vi "Acquire.vi"(8 "error in (no error)":errorcluster, 9 "DataNotifier":refnum<notifier>[](array[refnum]), 10 "DataQueues":refnum<queue>[](array[refnum]), 11 "Config In":T1 {"Hardware Configuration"."Lasers Configuration"."SettingValues"."785 Power" format="%.1f"; "Hardware Configuration"."Lasers Configuration"."SettingValues"."647 Power" format="%.1f"; "Hardware Configuration"."Lasers Configuration"."SettingValues"."561 Power" format="%.1f"; "Hardware Configuration"."Lasers Configuration"."SettingValues"."532 Power" format="%.1f"; "Hardware Configuration"."Lasers Configuration"."SettingValues"."488 Power" format="%.1f"; "Hardware Configuration"."Lasers Configuration"."SettingValues"."405 Power" format="%.1f"}) -> (0 "error out":errorcluster, 3 "Config Out":T1 {"Hardware Configuration"."Lasers Configuration"."SettingValues"."785 Power" format="%.1f"; "Hardware Configuration"."Lasers Configuration"."SettingValues"."647 Power" format="%.1f"; "Hardware Configuration"."Lasers Configuration"."SettingValues"."561 Power" format="%.1f"; "Hardware Configuration"."Lasers Configuration"."SettingValues"."532 Power" format="%.1f"; "Hardware Configuration"."Lasers Configuration"."SettingValues"."488 Power" format="%.1f"; "Hardware Configuration"."Lasers Configuration"."SettingValues"."405 Power" format="%.1f"})   [LabVIEW 2019, in "Acquisition.lvlib"]
doc: "Perform the acquisition. Replace the contents of this diagram with calls to acquisition hardware."
uses:
  Acquisition.lvlib
  Settings/Settings.ctl
  HardwareAdapter/Support/Hardware Configuration.ctl
  HardwareAdapter/Support/Camera Configuration.ctl
  D:/SDK/PMQI-LabViewSamples/Examples/Dependencies/PVCamNET.dll
  <vilib>/userdefined/High Color/IMAQdx.ctl
  E:/DevHardSoftware/MMicroscopy/HardwareAdapter/Lasers/Dependencies/Oxxius_Boxx.dll
  HardwareAdapter/Lasers/Dependencies/Oxxius_Boxx.dll
  Logging/Logging Configuration.ctl
  controls/UI Configuration.ctl
  Global.vi
  Logging/Logging.lvlib
  Settings/Settings.lvlib
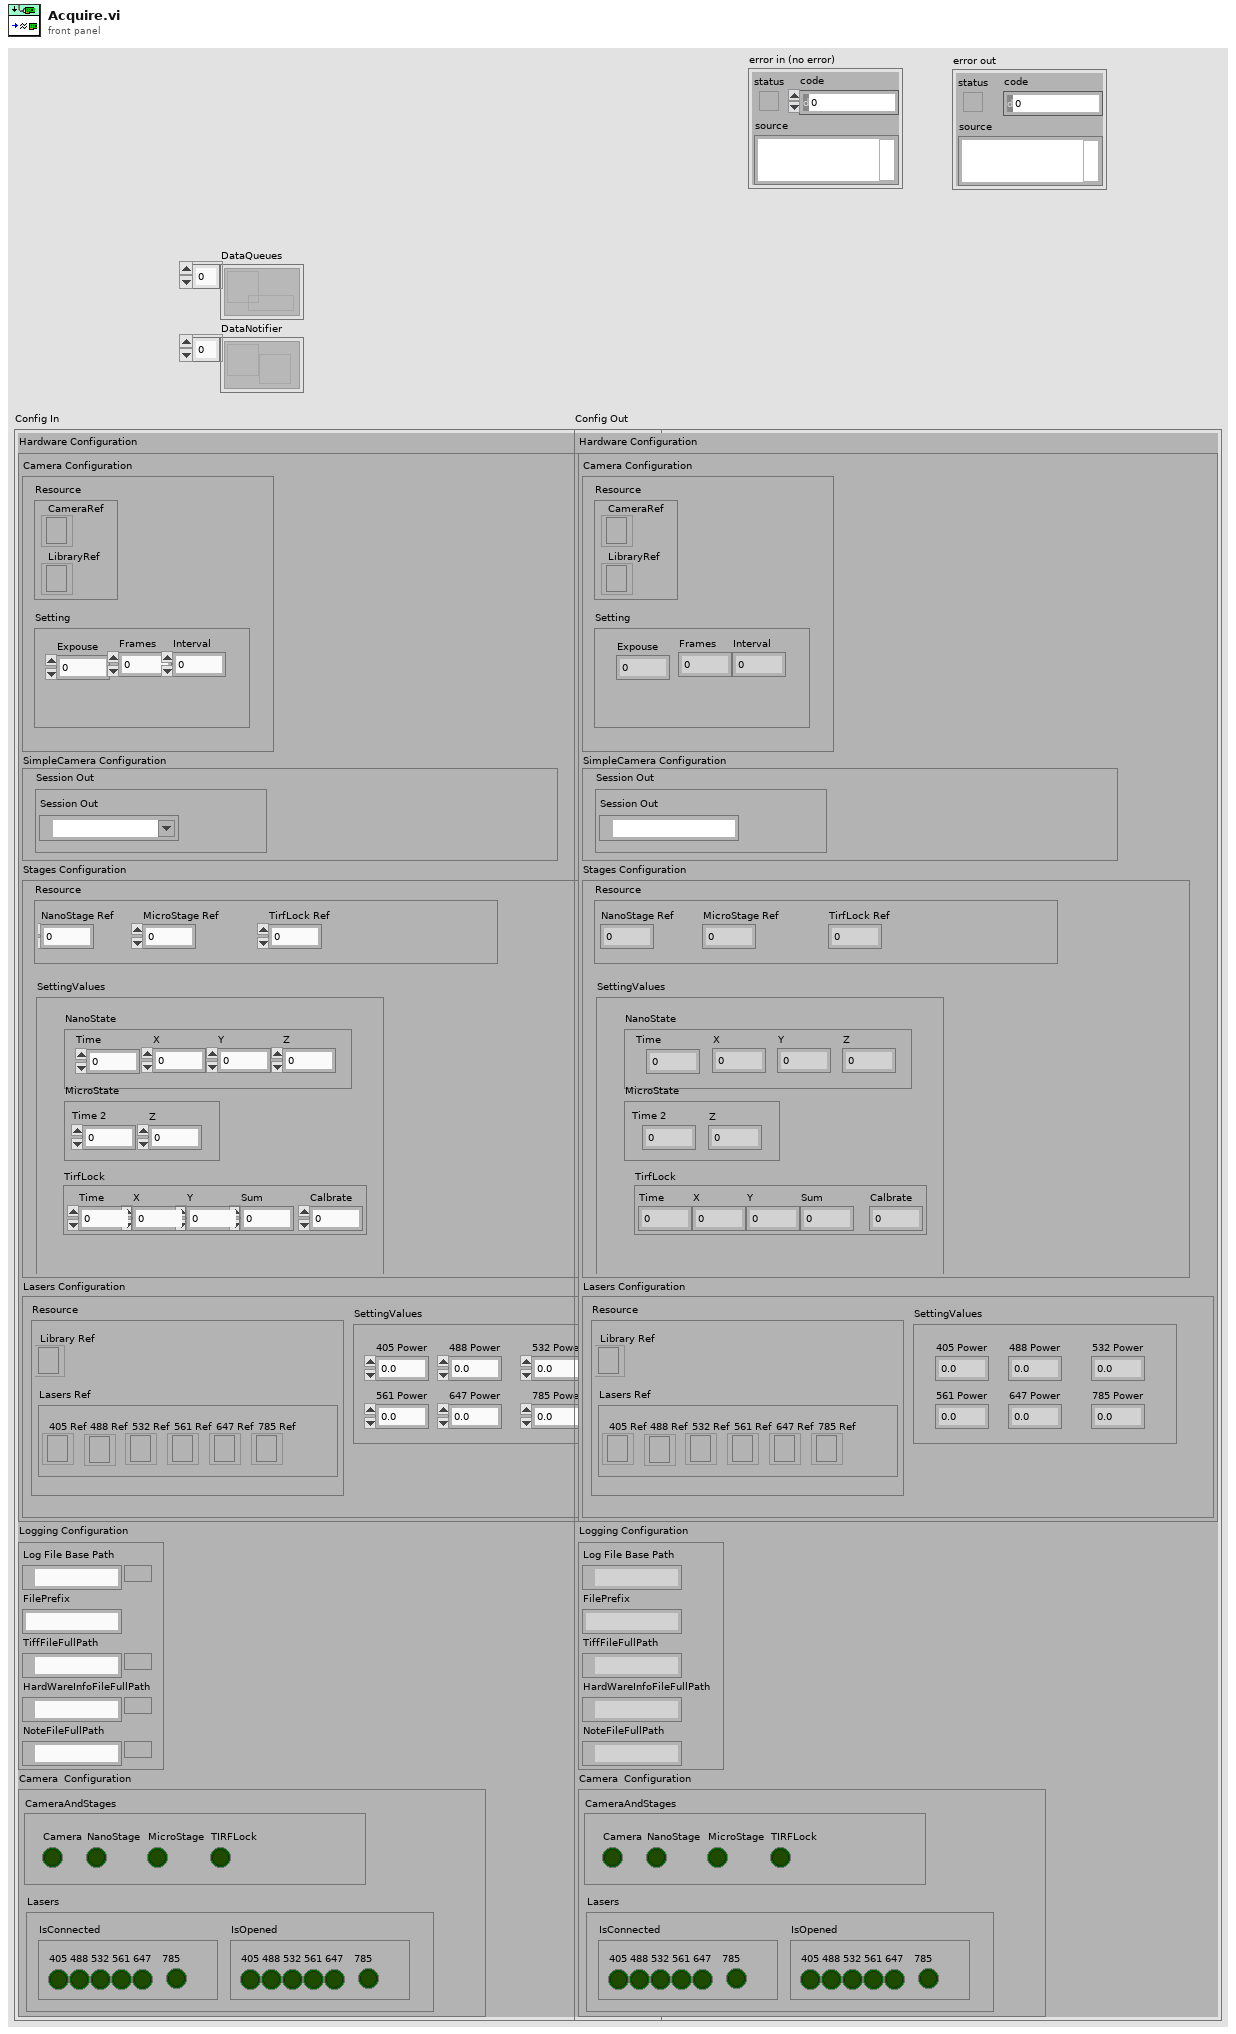
[diagram p1: front panel]
types:
  T1 = typedef "Settings.lvlib/Settings.ctl" = cluster{"Hardware Configuration":T2, "Logging Configuration":T5, "HardWare Status":cluster{"CameraAndStages":T6, "Lasers":cluster{"IsConnected":cluster{"405":bool, "488":bool, "532":bool, "561":bool, "647":bool, "785":bool}, "IsOpened":cluster{"405":bool, "488":bool, "532":bool, "561":bool, "647":bool, "785":bool}}}}
  T2 = typedef "Hardware Configuration.ctl" = cluster{"Camera Configuration":T3, "SimpleCamera Configuration":cluster{"Resource":cluster{"Session Out":T4}}, "Stages Configuration":cluster{"Resource":cluster{"NanoStage Ref":i32, "MicroStage Ref":i32, "TirfLock Ref":i32}, "SettingValues":cluster{"NanoState":cluster{"Time":dbl, "X":dbl, "Y":dbl, "Z":dbl}, "MicroState":cluster{"Time 2":dbl, "Z":dbl}, "TirfLock":cluster{"Time":dbl, "X":dbl, "Y":dbl, "Sum":dbl, "Calbrate":dbl}}}, "Lasers Configuration":cluster{"SettingValues":cluster{"405 Power":sgl, "488 Power":sgl, "532 Power":sgl, "561 Power":sgl, "647 Power":sgl, "785 Power":sgl}, "Resource":cluster{"Library Ref":refnum<k24>, "Lasers Ref":cluster{"405 Ref":refnum<k24>, "488 Ref":refnum<k24>, "532 Ref":refnum<k24>, "561 Ref":refnum<k24>, "647 Ref":refnum<k24>, "785 Ref":refnum<k24>}}}}
  T3 = typedef "Camera Configuration.ctl" = cluster{"Resource":cluster{"CameraRef":refnum<k24>, "LibraryRef":refnum<k24>}, "Setting":cluster{"Expouse":dbl, "Frames":dbl, "Interval":dbl}}
  T4 = typedef "IMAQdx.ctl" = refnum<k21>
  T5 = typedef "Logging.lvlib/Logging Configuration.ctl" = cluster{"Log File Base Path":path, "FilePrefix":string, "TiffFileFullPath":path, "HardWareInfoFileFullPath":path, "NoteFileFullPath":path}
  T6 = typedef "UI Configuration.ctl" = cluster{"Camera":bool, "NanoStage":bool, "MicroStage":bool, "TIRFLock":bool}
  T7 = typedef "ImageInfo.ctl" = cluster{"Time":dbl, "Image":T8, "Histogram":u32[], "MeanValue":dbl, "Min":u32, "Max":u32}
  T8 = typedef "IMAQ Image.ctl" = refnum<image>
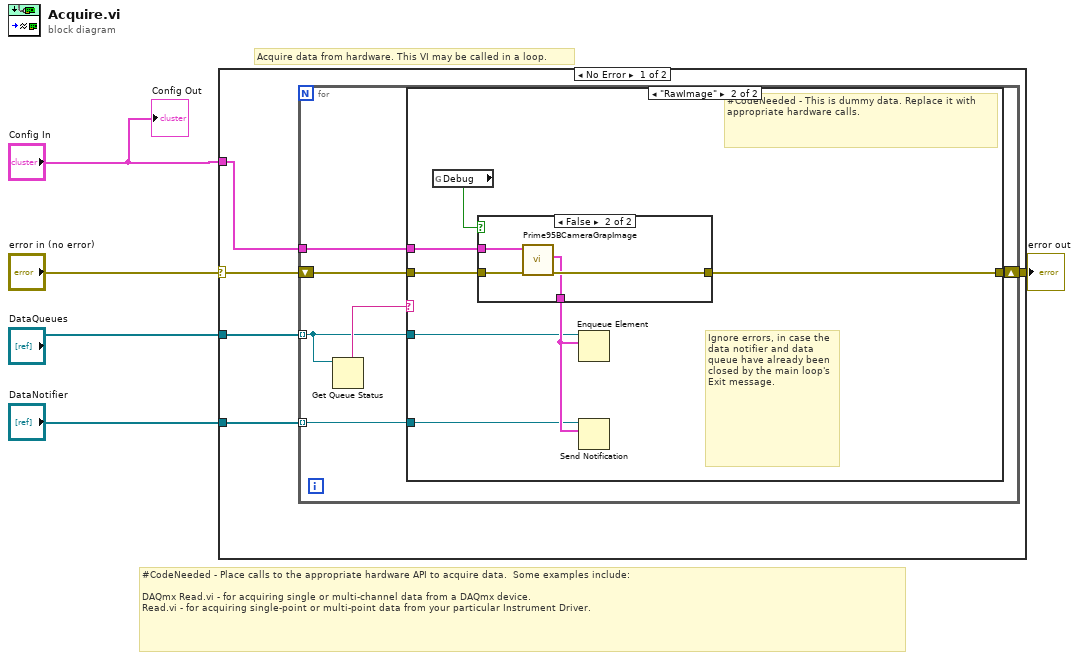
[diagram p0: block diagram]
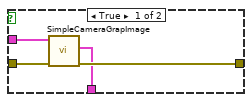
[diagram p3: hidden frame]
diagram:
  # "Acquire data from hardware. This VI may be called in a loop."
  # "#CodeNeeded - Place calls to the appropriate hardware API to acquire data.  Some examples include:\n\nDAQmx Read.vi - for acquiring single or multi-channel data from a DAQmx device.\nRead.vi - for acquiring single-point or multi-point data from your particular Instrument Driver."
  n1 = case shown="No Error" "error in (no error)" {
    selector: "error in (no error)" -> [w10 w33]
    tunnel: [w9 w33] -> w4
    tunnel: "DataNotifier" -> [w6 _]
    tunnel: "Config In" -> [w8 _]
    tunnel: "DataQueues" -> [w7 _]
    frame No Error {
      n2 = for {
        tunnel: w8 -> [w14]
        shift-right: [w15] -> w9
        shift-left: w10 -> [w16]
        tunnel: w7 -> [w11] mode=indexing
        tunnel: w6 -> [w12] mode=indexing
        n3 = Get Queue Status(queue=w11) -> (queue name=w13:string)  [unwired: 2 in, 7 out]
        n4 = case shown="\"RawImage\"" w13 {
          tunnel: w16 -> [w17 w24]
          tunnel: [w17 w23] -> w15
          tunnel: w14 -> [_ w22]
          tunnel: w11 -> [_ w18]
          tunnel: w12 -> [_ w19]
          frame "False", Default {
          }
          frame "RawImage" {
            # "Ignore errors, in case the data notifier and data queue have already been closed by the main loop's Exit message."
            # "#CodeNeeded - This is dummy data. Replace it with appropriate hardware calls."
            n5 = global read "Global.vi" "Debug"() -> (w20:bool)
            n6 = case shown="False" w20 {
              tunnel: w24 -> [w28 w32]
              tunnel: [w27 w31] -> w23
              tunnel: w22 -> [w26 w30]
              tunnel: [w25 w29] -> w21
              frame True {
                n7 = call "SimpleCameraGrapImage.vi"("error in (no error)"=w28, "Config In"=w26) -> ("error out"=w27:errorcluster, "RawImage"=w25:T7)  [unwired: 6 in, 1 out]
              }
              frame False {
                n8 = call "Prime95BCameraGrapImage.vi"("error in (no error)"=w32, "Config In"=w30) -> ("error out"=w31:errorcluster, "RawImage"=w29:T7)  [unwired: 6 in, 1 out]
              }
            }
            n9 = Enqueue Element(queue=w18, element=w21) -> ()  [unwired: 2 in, 3 out]
            n10 = Send Notification(notification=w21, notifier=w19) -> ()  [unwired: 1 in, 2 out]
          }
        }
      }
    }
    frame Error {
    }
  }
  "error out" <- w4
  "Config Out" <- "Config In"
